vi "Example One Stage.vi"() -> ()   [LabVIEW 2019]
uses:
  SMOs/Controller.LV/Controller.LV.lvclass
  <vilib>/Platform/TimedLoop/XDataNode/timing_clust.ctl
  <vilib>/Platform/TimedLoop/XDataNode/nitl_modes.ctl
  <vilib>/Platform/TimedLoop/XDataNode/wakeup.ctl
  <vilib>/platform/TimedLoop/XDataNode/XDataNode.xnode
  <vilib>/Platform/TimedLoop/XDataNode/XDNodeRunTimeDep.lvlib
panel:
  out "Desired Position\n[selected units]":dbl
  out "Encoder position \n[selected units]":dbl
  in  "Tab Control":enum32{"Motion", "Settings"}(tab)
  in  "Zero Output":bool
  in  "Go to Home":bool
  in  "Scan Right":bool
  in  "Scan Left":bool
  in  "Continue":bool
  in  "Stop":bool
  in  "Make Step Right":bool
  in  "Step Size \n[selected units]":dbl=1.0 format="%#.2f"
  in  "Make Step Left":bool
  in  "Desired Speed \n[1µm/s or 0,01deg /s]":dbl=10000.0 format="%#.4f"
  in  "Desired Position \n[selected units]":dbl format="%#.2f"
  in  "Find Index":bool
  in  "Reset":bool
  out "error out":errorcluster
  in  "Working Units":string(combo)="17453,292519943294"
  out "StatusBits":T1
  out "Status Info":T2
  in  "Axis Resolution":string(combo)="3.49065850399"
  in  "Axis Letter":string="X"
  in  "Baudrate":dbl=9600.0
  in  "COM Port":refnum<visa-resource-name>="COM4"
  out "Waveform Chart":dbl(graph)=-0.078
  in  "STOP PROGRAM":bool
  # "Visualization"
  # "Extra information"
  # "READ ME FIRST"
  # "Configuration"
  # "Stage 1"
  # "Driver 1"
  # "Stage 1"
  # "How to run:"
  # "BEFORE RUNNING:"
  # "1, Select COM Port"
  # "2. Select baudrate"
  # "3. For each axis:"
  # "3.1 Specify correct axis name (1 letter)"
  # "3.2 Specify correct resolution"
  # "4. Run VI"
  # "WHEN RUNNING, YOU HAVE TO FIRST PUSH \"FIND INDEX\" FOR EACH STAGE.\nThe stages will start moving and find its position. After that you can control the stages"
  # "NOTES: Do this only the first time"
  # "1. Replace the settings_default.txt file with\nthe file we provided on a USB stick."
  # "2.    Make sure there are no comments in the\nsettings_default.txt file. ONLY lines like: \"X:DPOS=100\" so NO \"%\" in front or at the end of the line."
  # "Position Information"
  # "STOP BUTTON"
  # "3.  In your settings_default.txt file:\nEvery line that contains SSPD or MSPD: multiply that value with:\n - 1000 for a lineair stage \n - 100 for a rotating stage"
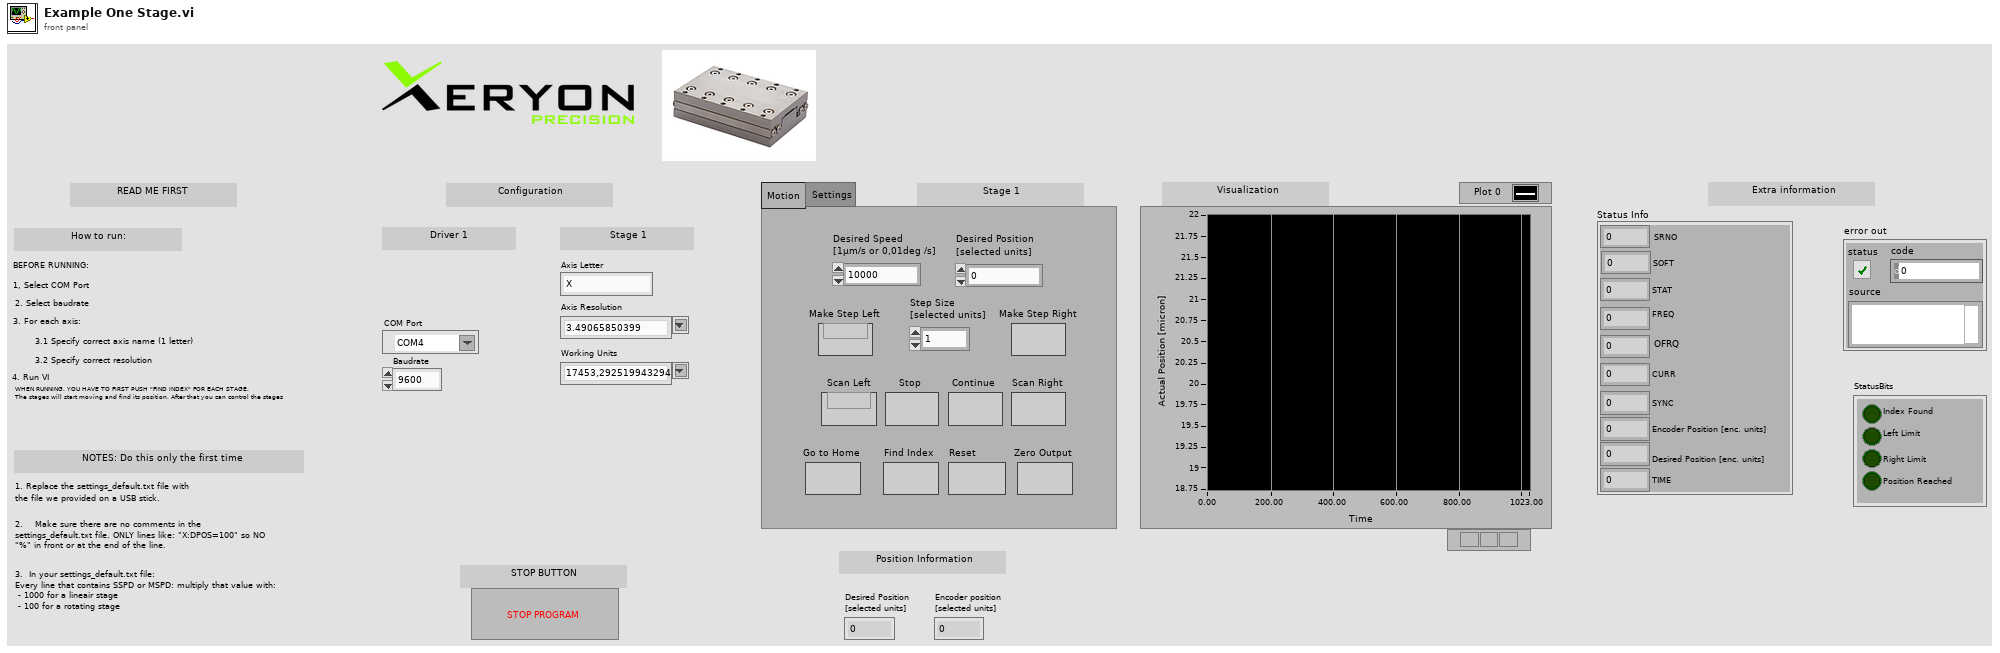
[diagram p1: front panel]
types:
  T1 = cluster{"Index Found":bool, "Left Limit":bool, "Right Limit":bool, "Position Reached":bool}
  T2 = cluster{"SRNO":dbl, "SOFT":dbl, "STAT":dbl, "FREQ":dbl, "OFRQ":dbl, "CURR":dbl, "SYNC":dbl, "Encoder Position [enc. units]":dbl, "Desired Position [enc. units]":dbl, "TIME":dbl}
  T3 = typedef "XDNodeRunTimeDep.lvlib/timing_clust.ctl" = cluster{"Expected End [f-1]":u64, "Actual End [f-1]":u64, "Finished Late? [f-1]":bool, "Expected End [i-1]":u64, "Actual End [i-1]":u64, "Finished Late? [i-1]":bool, "Expected Start [i]":u64, "Actual Start [i]":u64, "Expected Start [f]":u64, "Actual Start [f]":u64, "Source Name":string, "Structure Name":string, "Period":i64, "Deadline":i64, "Offset":i64, "Start":i64, "Priority":i32, "Timeout":i32, "Mode":T4, "Wakeup Reason":T5, "Error":errorcluster, "Source Type":string, "Secondary Source Type":string, "Global End Time":u64, "Global Start Time":u64, "Frame Duration":u64, "Iteration Duration":u64, "Assigned CPU":i32, "I/O Scan Engine Mode":u32}
  T4 = typedef "XDNodeRunTimeDep.lvlib/nitl_modes.ctl" = enum32{"No Change", "Process missed periods, maintain original phase", "Discard missed periods, maintain original phase", "Process missed periods, ignore original phase", "Discard missed periods, ignore original phase"}
  T5 = typedef "XDNodeRunTimeDep.lvlib/wakeup.ctl" = enum32{"Normal", "Aborted", "Asynchronous wakeup", "Timing source error", "Timed loop error", "Timeout"}
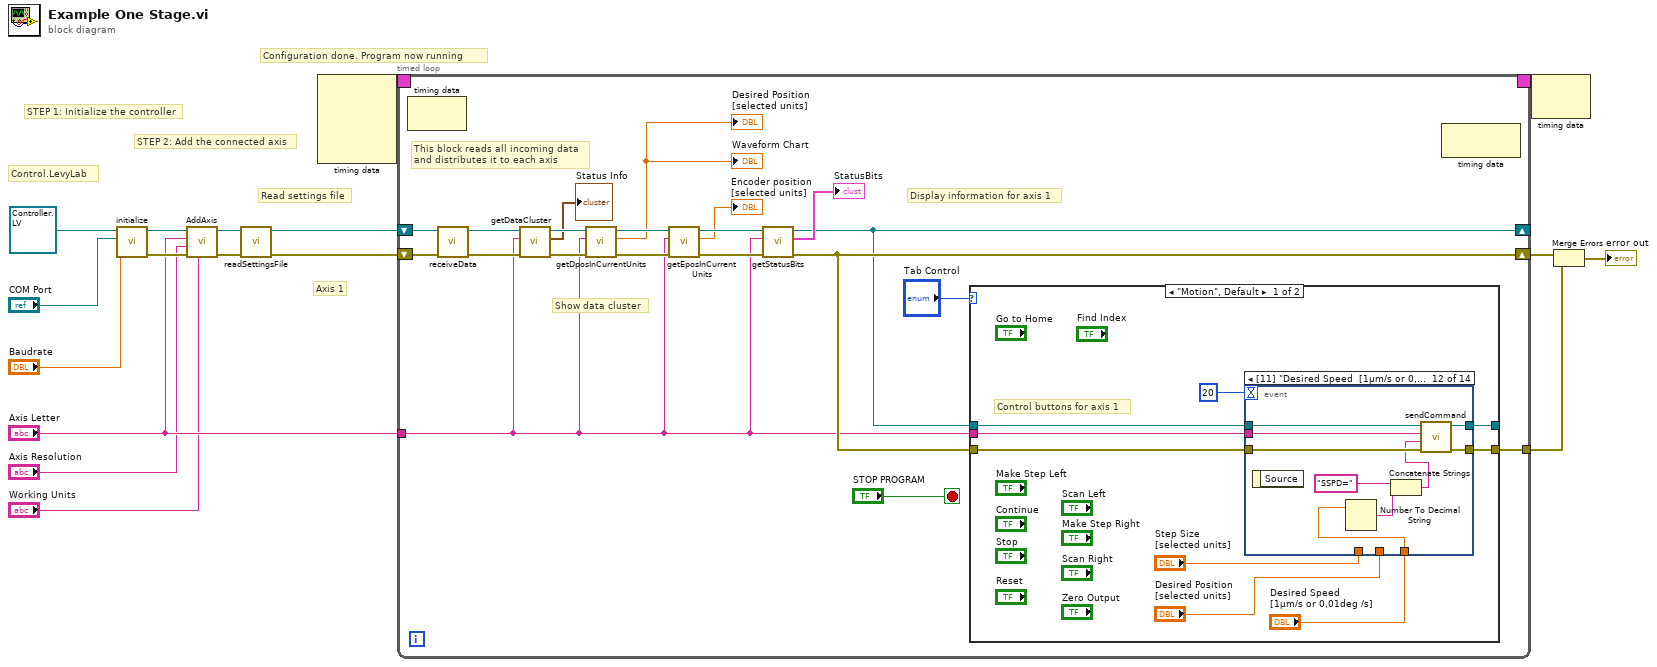
[diagram p0: block diagram]
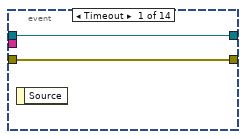
[diagram p2: hidden frame]
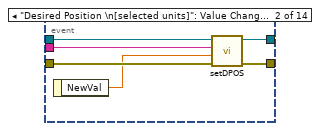
[diagram p3: hidden frame]
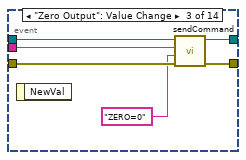
[diagram p4: hidden frame]
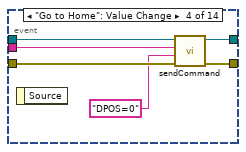
[diagram p5: hidden frame]
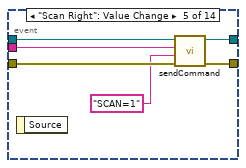
[diagram p6: hidden frame]
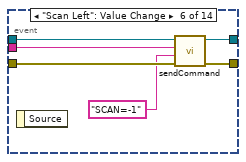
[diagram p7: hidden frame]
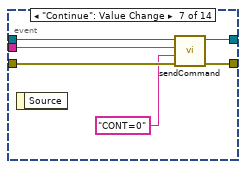
[diagram p8: hidden frame]
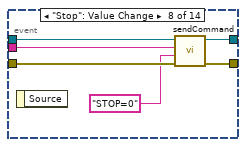
[diagram p9: hidden frame]
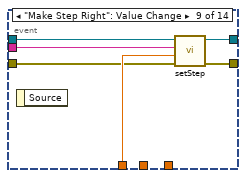
[diagram p10: hidden frame]
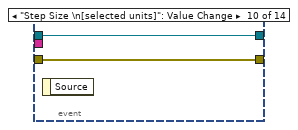
[diagram p11: hidden frame]
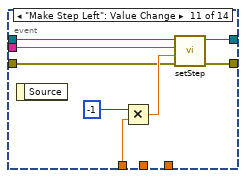
[diagram p12: hidden frame]
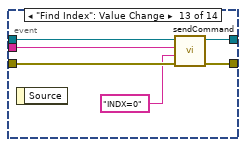
[diagram p13: hidden frame]
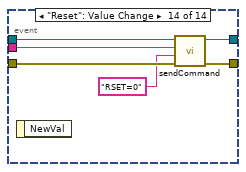
[diagram p14: hidden frame]
diagram:
  # "Control.LevyLab"
  # "Axis 1"
  # "Configuration done. Program now running"
  # "Read settings file"
  # "STEP 2: Add the connected axis"
  # "STEP 1: Initialize the controller"
  n1 = call-dynamic "initialize.vi"("Baudrate"="Baudrate", "COM Port"="COM Port", "Controller in"=refnum<class "Controller.LV.lvclass"> refnum ("Controller.LV.lvclass")) -> ("error out"=w16:errorcluster, "Controller out"=w17:refnum<class "Controller.LV.lvclass">)  [unwired: 7 in]
  n2 = call-dynamic "AddAxis.vi"("Units"="Working Units", "error in (no error)"=w16, "Encoder Resolution"="Axis Resolution", "Axis Letter"="Axis Letter", "Controller.LV in"=w17) -> ("error out"=w11:errorcluster, "Controller.LV out"=w13:refnum<class "Controller.LV.lvclass">)  [unwired: 5 in]
  n3 = call-dynamic "readSettingsFile.vi"("error in (no error)"=w11, "Controller.LV in"=w13) -> ("error out"=w10:errorcluster, "Controller.LV out"=w12:refnum<class "Controller.LV.lvclass">)  [unwired: 8 in]
  n4 = node-c288() -> (w5:T3)  [unwired: 4 in]
  n5 = timed-loop {
    shift-right: [w19] -> _
    shift-left: w12 -> [w37]
    tunnel: "Axis Letter" -> [w18]
    shift-right: [w23] -> w3
    shift-left: w10 -> [w26]
    timing: w5 -> [_]
    timing-out: [_] -> w4
    tunnel: [w22] -> w2
    stop <- "STOP PROGRAM" stop-if-true
    # "Display information for axis 1"
    # "Show data cluster"
    # "This block reads all incoming data\nand distributes it to each axis"
    n6 = node-c288() -> ()  [unwired: 1 in, 1 out]
    n7 = call-dynamic "receiveData.vi"("error in (no error)"=w26, "Controller.LV in"=w37) -> ("error out"=w35:errorcluster, "Controller.LV out"=w36:refnum<class "Controller.LV.lvclass">)  [unwired: 8 in]
    n8 = call-dynamic "getDataCluster.vi"("error in (no error)"=w35, "Axis Letter"=w18, "Controller in"=w36) -> ("error out"=w30:errorcluster, "Information"=→"Status Info":T2, "Controller out"=w33:refnum<class "Controller.LV.lvclass">)  [unwired: 6 in]
    n9 = call-dynamic "getDposInCurrentUnits.vi"("error in (no error)"=w30, "Axis Letter"=w18, "Controller in"=w33) -> ("error out"=w29:errorcluster, "DPOS In Current Units"=→"Waveform Chart" →"Desired Position\n[selected units]":dbl, "Controller out"=w32:refnum<class "Controller.LV.lvclass">)  [unwired: 6 in]
    n10 = call-dynamic "getEposInCurrentUnits.vi"("error in (no error)"=w29, "Axis Letter"=w18, "Controller in"=w32) -> ("error out"=w28:errorcluster, "EPOS In Current Units"=→"Encoder position \n[selected units]":dbl, "Controller out"=w31:refnum<class "Controller.LV.lvclass">)  [unwired: 6 in]
    n11 = call-dynamic "getStatusBits.vi"("error in (no error)"=w28, "Axis Letter"=w18, "Controller in"=w31) -> ("error out"=w23:errorcluster, "StatusBits"=→"StatusBits":T1, "Controller out"=w19:refnum<class "Controller.LV.lvclass">)  [unwired: 6 in]
    n12 = case shown="\"Motion\", Default" "Tab Control" {
      tunnel: w19 -> [w48 w130]
      tunnel: w23 -> [w47 w131]
      tunnel: [w46 w130] -> _
      tunnel: [w45 w131] -> w22
      tunnel: w18 -> [w43 _]
      frame "Motion", Default {
        # "Control buttons for axis 1"
        n13 = event shown="[11] \"Desired Speed  [1µm/s or 0,01deg /s]\": Value Change" {
          selector: _ -> [_ _ _ _ _ _ _ _ _ _ _ _ _ _]
          dyn-events: _ -> [_ _ _ _ _ _ _ _ _ _ _ _ _ _]
          timeout: 20 -> [_ _ _ _ _ _ _ _ _ _ _ _ _ _]
          tunnel: w48 -> [w50 w56 w62 w68 w74 w80 w86 w92 w96 w100 w106 w117 w123 w129]
          tunnel: w47 -> [w49 w55 w60 w66 w72 w78 w84 w90 w97 w99 w103 w115 w122 w128]
          tunnel: [w50 w53 w58 w64 w70 w76 w82 w88 w94 w100 w101 w110 w120 w126] -> w46
          tunnel: [w49 w54 w59 w65 w71 w77 w83 w89 w93 w99 w102 w111 w121 w125] -> w45
          tunnel: w43 -> [_ w51 w61 w67 w73 w79 w85 w91 w95 _ w105 w116 w119 w127]
          tunnel: "Step Size \n[selected units]" -> [_ _ _ _ _ _ _ _ w98 _ w107 _ _ _]
          tunnel: "Desired Position \n[selected units]" -> [_ _ _ _ _ _ _ _ _ _ _ _ _ _]
          tunnel: "Desired Speed \n[1µm/s or 0,01deg /s]" -> [_ _ _ _ _ _ _ _ _ _ _ w114 _ _]
          event Timeout {
            n14 = event-data() -> ()  [unwired: 1 in, 1 out]
          }
          event "Desired Position \n[selected units]": Value Change {
            n15 = event-data() -> ("NewVal"=w52:dbl)  [unwired: 1 in]
            n16 = call-dynamic "setDPOS.vi"("error in (no error)"=w55, "DPOS In Current Units"=w52, "Axis Letter"=w51, "Controller in"=w56) -> ("error out"=w54:errorcluster, "Controller out"=w53:refnum<class "Controller.LV.lvclass">)  [unwired: 6 in]
          }
          event "Zero Output": Value Change {
            n17 = event-data() -> ()  [unwired: 1 in, 1 out]
            n18 = call-dynamic "sendCommand.vi"("error in (no error)"=w60, "Command"="ZERO=0", "Axis Letter"=w61, "Controller in"=w62) -> ("error out"=w59:errorcluster, "Controller out"=w58:refnum<class "Controller.LV.lvclass">)  [unwired: 6 in]
          }
          event "Go to Home": Value Change {
            n19 = event-data() -> ()  [unwired: 1 in, 1 out]
            n20 = call-dynamic "sendCommand.vi"("error in (no error)"=w66, "Command"="DPOS=0", "Axis Letter"=w67, "Controller in"=w68) -> ("error out"=w65:errorcluster, "Controller out"=w64:refnum<class "Controller.LV.lvclass">)  [unwired: 6 in]
          }
          event "Scan Right": Value Change {
            n21 = event-data() -> ()  [unwired: 1 in, 1 out]
            n22 = call-dynamic "sendCommand.vi"("error in (no error)"=w72, "Command"="SCAN=1", "Axis Letter"=w73, "Controller in"=w74) -> ("error out"=w71:errorcluster, "Controller out"=w70:refnum<class "Controller.LV.lvclass">)  [unwired: 6 in]
          }
          event "Scan Left": Value Change {
            n23 = event-data() -> ()  [unwired: 1 in, 1 out]
            n24 = call-dynamic "sendCommand.vi"("error in (no error)"=w78, "Command"="SCAN=-1", "Axis Letter"=w79, "Controller in"=w80) -> ("error out"=w77:errorcluster, "Controller out"=w76:refnum<class "Controller.LV.lvclass">)  [unwired: 6 in]
          }
          event "Continue": Value Change {
            n25 = event-data() -> ()  [unwired: 1 in, 1 out]
            n26 = call-dynamic "sendCommand.vi"("error in (no error)"=w84, "Command"="CONT=0", "Axis Letter"=w85, "Controller in"=w86) -> ("error out"=w83:errorcluster, "Controller out"=w82:refnum<class "Controller.LV.lvclass">)  [unwired: 6 in]
          }
          event "Stop": Value Change {
            n27 = event-data() -> ()  [unwired: 1 in, 1 out]
            n28 = call-dynamic "sendCommand.vi"("error in (no error)"=w90, "Command"="STOP=0", "Axis Letter"=w91, "Controller in"=w92) -> ("error out"=w89:errorcluster, "Controller out"=w88:refnum<class "Controller.LV.lvclass">)  [unwired: 6 in]
          }
          event "Make Step Right": Value Change {
            n29 = event-data() -> ()  [unwired: 1 in, 1 out]
            n30 = call-dynamic "setStep.vi"("error in (no error)"=w97, "Step Value"=w98, "Axis Letter"=w95, "Controller in"=w96) -> ("error out"=w93:errorcluster, "Controller out"=w94:refnum<class "Controller.LV.lvclass">)  [unwired: 6 in]
          }
          event "Step Size \n[selected units]": Value Change {
            n31 = event-data() -> ()  [unwired: 1 in, 1 out]
          }
          event "Make Step Left": Value Change {
            n32 = event-data() -> ()  [unwired: 1 in, 1 out]
            n33 = Multiply(x=-1, y=w107) -> (x*y=w104:dbl)
            n34 = call-dynamic "setStep.vi"("error in (no error)"=w103, "Step Value"=w104, "Axis Letter"=w105, "Controller in"=w106) -> ("error out"=w102:errorcluster, "Controller out"=w101:refnum<class "Controller.LV.lvclass">)  [unwired: 6 in]
          }
          event "Desired Speed \n[1µm/s or 0,01deg /s]": Value Change {
            n35 = event-data() -> ()  [unwired: 1 in, 1 out]
            n36 = Number To Decimal String(number=w114) -> (decimal integer string=w112:string)  [unwired: 1 in]
            n37 = Concatenate Strings("SSPD=", w112) -> (w109:string)
            n38 = call-dynamic "sendCommand.vi"("error in (no error)"=w115, "Command"=w109, "Axis Letter"=w116, "Controller in"=w117) -> ("error out"=w111:errorcluster, "Controller out"=w110:refnum<class "Controller.LV.lvclass">)  [unwired: 6 in]
          }
          event "Find Index": Value Change {
            n39 = event-data() -> ()  [unwired: 1 in, 1 out]
            n40 = call-dynamic "sendCommand.vi"("error in (no error)"=w122, "Command"="INDX=0", "Axis Letter"=w119, "Controller in"=w123) -> ("error out"=w121:errorcluster, "Controller out"=w120:refnum<class "Controller.LV.lvclass">)  [unwired: 6 in]
          }
          event "Reset": Value Change {
            n41 = event-data() -> ()  [unwired: 1 in, 1 out]
            n42 = call-dynamic "sendCommand.vi"("error in (no error)"=w128, "Command"="RSET=0", "Axis Letter"=w127, "Controller in"=w129) -> ("error out"=w125:errorcluster, "Controller out"=w126:refnum<class "Controller.LV.lvclass">)  [unwired: 6 in]
          }
        }
      }
      frame "Settings" {
      }
    }
    n43 = node-c288() -> ()  [unwired: 1 in, 1 out]
  }
  n44 = node-c288(w4) -> ()  [unwired: 1 out]
  n45 = Merge Errors(w3, w2) -> (→"error out":errorcluster)
